vi "main.vi"() -> ()   [LabVIEW 2010]
uses:
  components_cluster.ctl
  components/Clock/GenericClock/GenericClock/GenericClock.lvclass
  components/SignalWriter/GenericSignalWriter/GenericSignalWriter/GenericSignalWriter.lvclass
  components/SignalReader/GenericSignalReader/GenericSignalReader/GenericSignalReader.lvclass
  configuration_cluster.ctl
  common/clusters/plugin_specification.ctl
  main/labview_source/type_definitions/enumerations/run_mode_enum.ctl
  <vilib>/Utility/file.llb/Write To Spreadsheet File (DBL).vi
  <vilib>/Analysis/2dsp.llb/1D Cross Correlation (DBL).vi
  common/classes/GenericComponent/GenericComponent/GenericComponent.lvclass
  <vilib>/Analysis/NI_AALPro.lvlib
panel:
  in  "normalization":enum32{"none", "unbiased", "biased"}(ring)
  in  "algorithm":enum32{"direct", "frequency domain"}(ring)
  out "phase shift":dbl[unit]
  in  "saveButton":bool
  out "cross correlation":dbl[](graph)
  in  "analyseButton":bool
  in  "channel index":i32
  out "data":dbl[](graph)
  in  "read block size":i32=16000
  in  "specifyClockButton":bool
  in  "specifyReaderButton":bool
  in  "sampling rate":dbl[unit]=20000.0
  in  "duration":dbl[unit]=1.0
  in  "specifyWriterButton":bool
  in  "stopButton":bool
  in  "startButton":bool
  in  "amplitude":dbl=1.0
  in  "frequency":dbl[unit]=10.0
  # "Amplitude and phase shift analyser"
  # "command values"
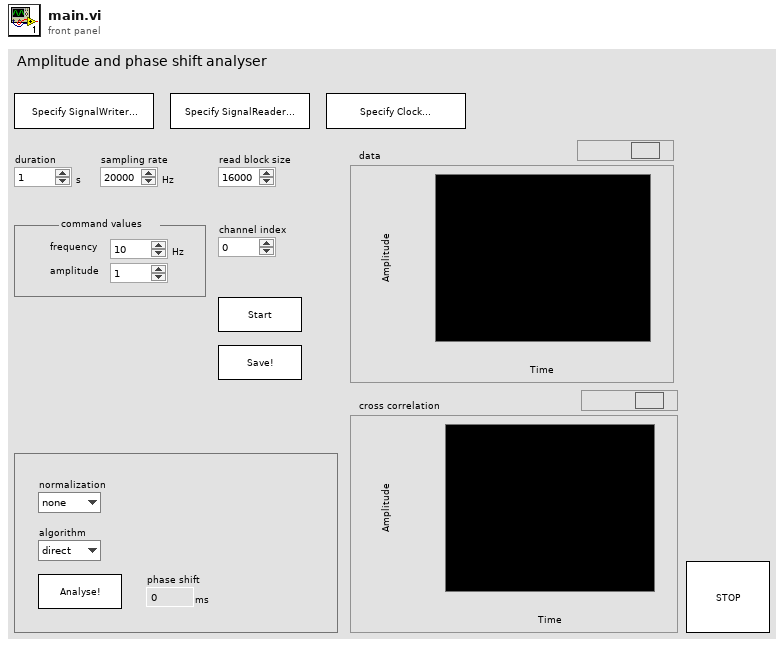
[diagram p1: front panel]
types:
  T1 = typedef "configuration_cluster.ctl" = cluster{"clock":T2, "writer":T2, "reader":T2}
  T2 = typedef "plugin_specification.ctl" = cluster{"class path":string, "configuration":string, "label":string, "settings name":string}
  T3 = typedef "components_cluster.ctl" = cluster{"clock":refnum<class "GenericClock.lvclass">, "writer":refnum<class "GenericSignalWriter.lvclass">, "reader":refnum<class "GenericSignalReader.lvclass">}
  T4 = typedef "run_mode_enum.ctl" = enum16{"focus mode", "single sweep mode", "experiment mode"}
  T5 = typedef "XComponentSpecification.xctl/data.ctl" = cluster{"class path":string, "configuration":string, "label":string, "settings name":string}
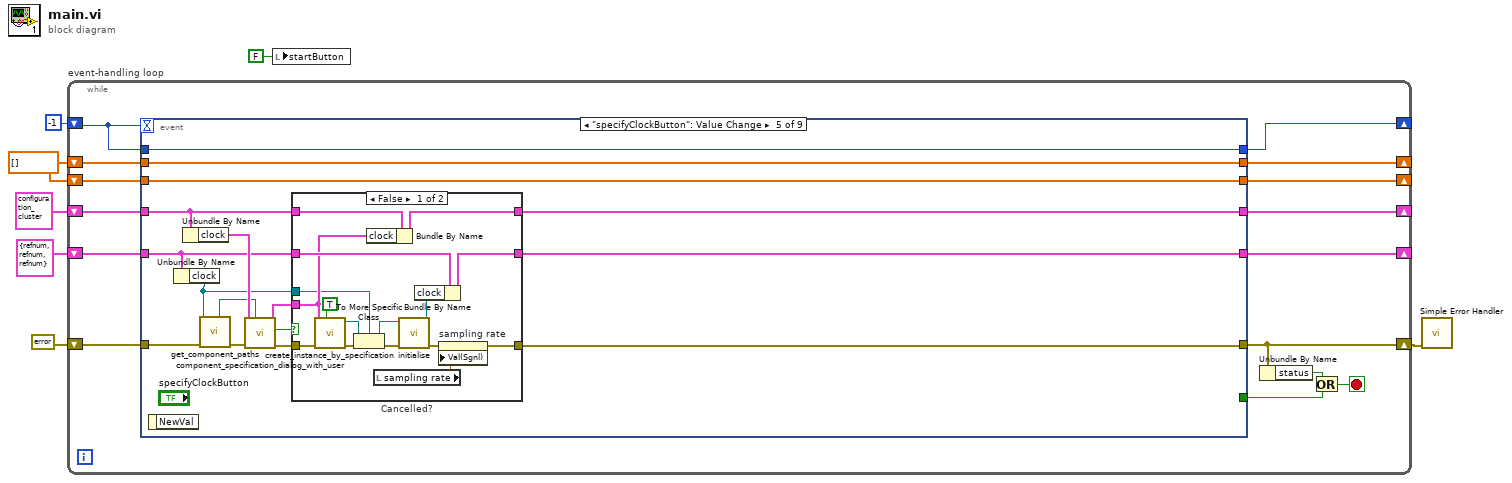
[diagram p0: block diagram]
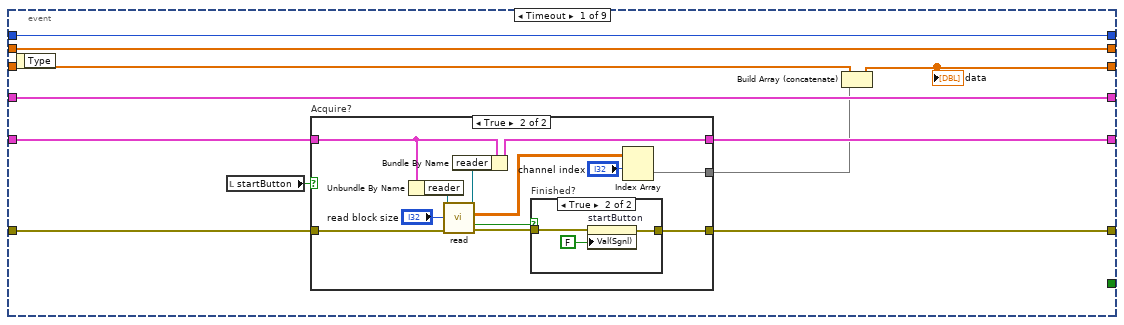
[diagram p2: hidden frame]
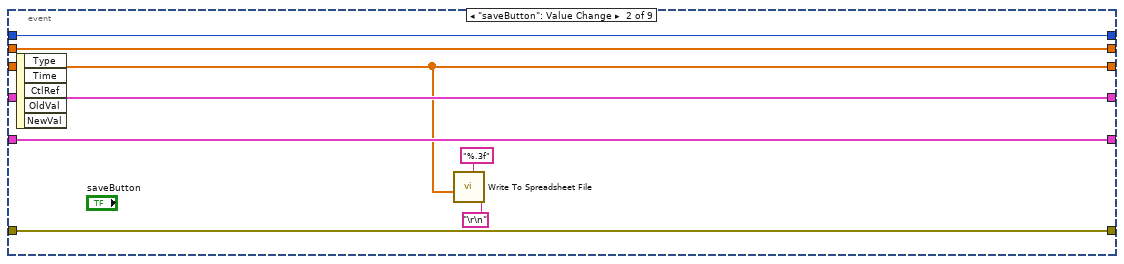
[diagram p5: hidden frame]
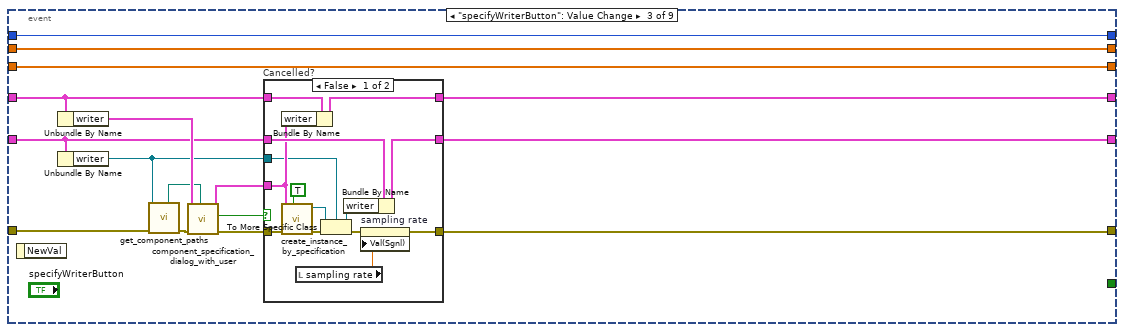
[diagram p6: hidden frame]
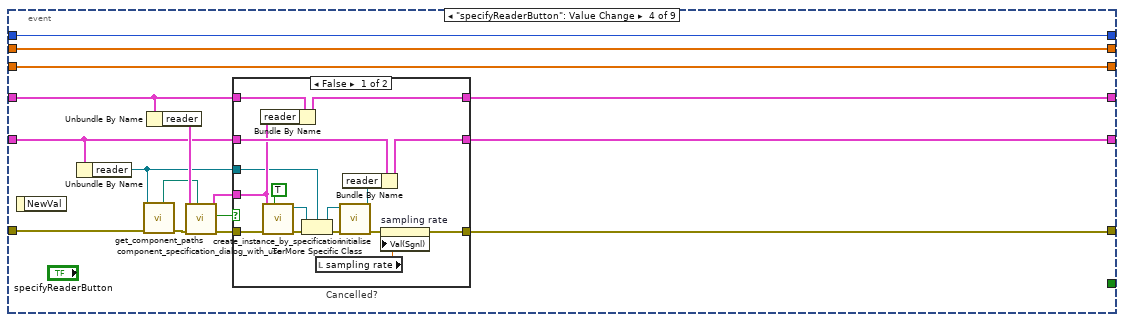
[diagram p8: hidden frame]
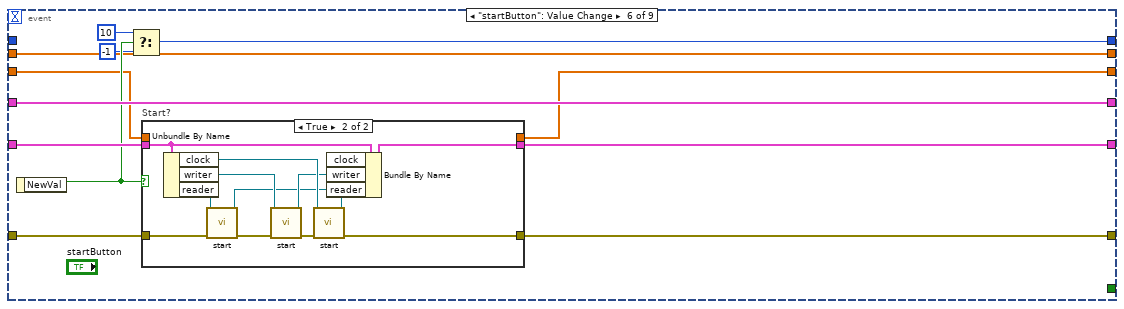
[diagram p11: hidden frame]
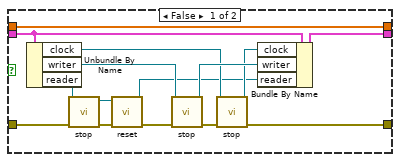
[diagram p12: hidden frame]
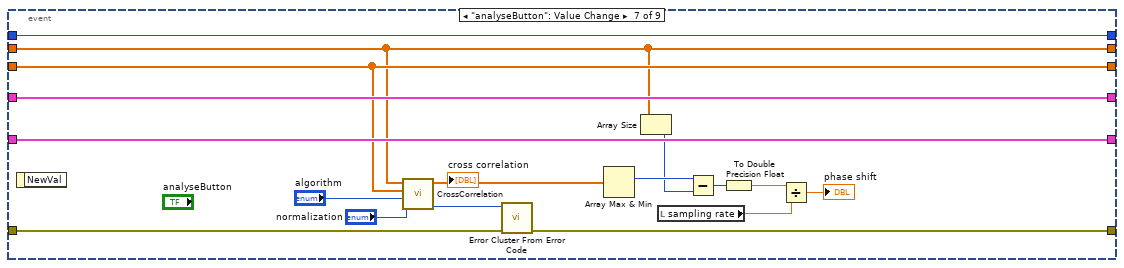
[diagram p13: hidden frame]
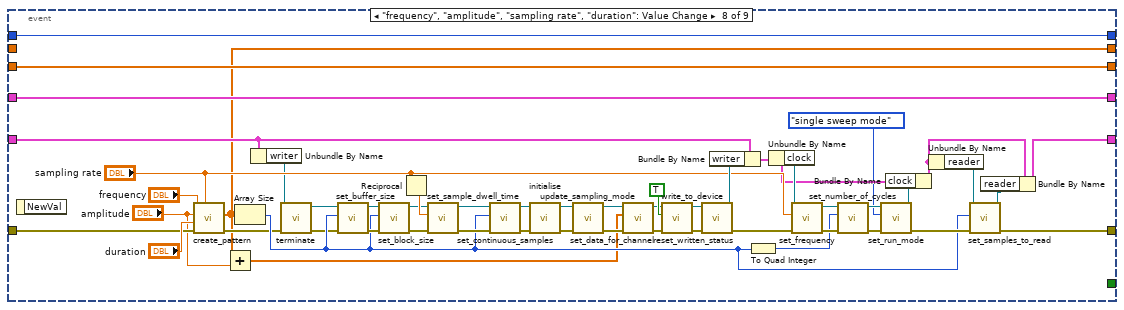
[diagram p14: hidden frame]
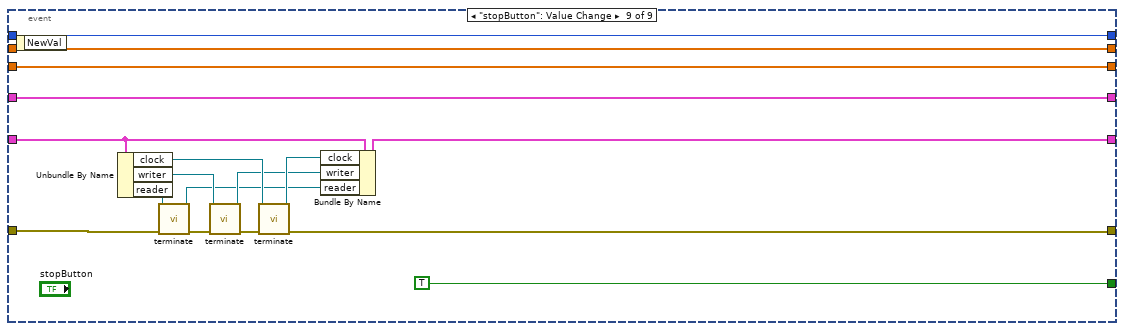
[diagram p15: hidden frame]
diagram:
  w1 = dbl[] [] ("pattern values")
  n1 = while "event-handling loop" {
    shift-right: [w21] -> w7
    shift-left: errorcluster {"status"=FALSE, "code"=0, "source"=""} ("error in (no error)") -> [w22]
    shift-right: [w16] -> _
    shift-left: T3 {"clock"=refnum, "writer"=refnum, "reader"=refnum} ("components") -> [w17]
    shift-right: [w15] -> _
    shift-left: -1 -> [w12]
    shift-right: [w13] -> _
    shift-left: T1 {"clock"={"class path"="", "configuration"="", "label"="", "settings name"=""}, "writer"={"class path"="", "configuration"="", "label"="", "settings name"=""}, "reader"={"class path"="", "configuration"="", "label"="", "settings name"=""}} ("configuration") -> [w14]
    shift-right: [w11] -> _
    shift-left: w1 -> [w10]
    shift-right: [w8] -> _
    shift-left: w1 -> [w9]
    stop <- w19 stop-if-true
    n2 = event shown="[4] \"specifyClockButton\": Value Change" {
      selector: _ -> [_ _ _ _ _ _ _ _ _]
      dyn-events: _ -> [_ _ _ _ _ _ _ _ _]
      timeout: w12 -> [_ _ _ _ _ _ _ _ _]
      tunnel: w22 -> [w30 w55 w64 w98 w132 w174 w213 w248 w284]
      tunnel: [w27 w55 w73 w104 w139 w173 w212 w237 w280] -> w21
      tunnel: [_ _ _ _ _ _ _ _ TRUE] -> w18
      tunnel: w17 -> [w32 w59 w65 w95 w131 w172 w218 w246 w277]
      tunnel: [w31 w59 w71 w103 w138 w171 w218 w233 w276] -> w16
      tunnel: [w28 w58 w75 w108 w143 w169 w211 w269 w285] -> w15
      tunnel: w14 -> [w33 w57 w69 w101 w137 w170 w217 w245 w272]
      tunnel: [w33 w57 w68 w102 w136 w170 w217 w245 w272] -> w13
      tunnel: w12 -> [w28 w58 w75 w108 w143 _ w211 w269 w285]
      tunnel: [w26 w56 w61 w94 w129 w165 w209 w221 w271] -> w11
      tunnel: w10 -> [w26 w56 w61 w94 w129 w165 w209 _ w271]
      tunnel: w9 -> [w25 w54 w60 w93 w128 w163 w216 w227 w270]
      tunnel: [w23 w54 w60 w93 w128 w164 w216 w227 w270] -> w8
      event Timeout {
        n3 = event-data() -> ()  [unwired: 1 in, 1 out]
        n4 = local read "startButton"() -> (w29:bool)
        n5 = case "Acquire?" shown="True" w29 {
          tunnel: w32 -> [w35 w46]
          tunnel: [w35 w45] -> w31
          tunnel: w30 -> [w34 w44]
          tunnel: [w34 w40] -> w27
          tunnel: [_ w36] -> w24
          frame False {
          }
          frame True {
            n6 = Unbundle By Name(w46) -> ("reader"=w43:refnum<class "GenericSignalReader.lvclass">)
            n7 = call-dynamic "read.vi"("error in (no error)"=w44, "block size"="read block size", "SignalReader in"=w43) -> ("error out"=w41:errorcluster, "finished?"=w39:bool, "signals read"=w38:dbl[][], "SignalReader out"=w47:refnum<class "GenericSignalReader.lvclass">)  [unwired: 4 in, 1 out]
            n8 = Bundle By Name(cluster=w46, "reader"=w47) -> (w45:T3)
            n9 = case "Finished?" shown="True" w39 {
              tunnel: w41 -> [w48 w51]
              tunnel: [w48 w50] -> w40
              frame False {
              }
              frame True {
                n10 = property on="startButton" class="Bool (strict)"(error in=w51, "Val(Sgnl)"=FALSE ("Value (Signaling)")) -> (error out=w50:errorcluster)  [unwired: 1 in, 1 out]
              }
            }
            n11 = Index Array(array=w38, index (row)="channel index") -> (element=w36:dbl[])  [unwired: 1 in]
          }
        }
        n12 = Build Array (concatenate)(w25, w24) -> (w23:dbl[])
        "data" <- w23
      }
      event "saveButton": Value Change {
        n13 = event-data() -> ()  [unwired: 1 in, 5 out]
        n14 = call-poly <vilib>:"Write To Spreadsheet File.vi"("delimiter (\\t)"="\r\n", "format (%.3f)"="%.3f", "1D data"=w54) -> ()  [unwired: 5 in, 1 out]
      }
      event "specifyWriterButton": Value Change {
        n15 = event-data() -> ()  [unwired: 1 in, 1 out]
        n16 = Unbundle By Name(w69) -> ("writer"=w67:T2)
        n17 = Unbundle By Name(w65) -> ("writer"=w62:refnum<class "GenericSignalWriter.lvclass">)
        n18 = call-dynamic "get_component_paths.vi"("error in (no error)"=w64, "GenericComponent in"=w62) -> ("error out"=w63:errorcluster, "component type directory"=w66:path)  [unwired: 4 in, 4 out]
        n19 = call "component_specification_dialog_with_user.vi"("start path"=w66, "error in (no error)"=w63, "component specification in"=w67) -> ("error out"=w74:errorcluster, "cancelled?"=w72:bool, "component specification out"=w70:T5)  [unwired: 6 in]
        n20 = case "Cancelled?" shown="False" w72 {
          tunnel: w74 -> [w84 w92]
          tunnel: [w88 w92] -> w73
          tunnel: [w87 w91] -> w71
          tunnel: w65 -> [w79 w91]
          tunnel: w70 -> [w77 _]
          tunnel: w69 -> [w86 w90]
          tunnel: [w85 w90] -> w68
          tunnel: w62 -> [w76 _]
          frame False {
            n21 = Bundle By Name(cluster=w86, "writer"=w77) -> (w85:T1)
            n22 = call "create_instance_by_specification.vi"("call constructor?"=TRUE, "error in (no error)"=w84, "component specification"=w77) -> ("error out"=w81:errorcluster, "GenericPlugin out"=w82:refnum<class "GenericComponent.lvclass">)  [unwired: 6 in, 1 out]
            n23 = local read "sampling rate"() -> (w89:dbl[unit])
            n24 = To More Specific Class(target class=w76, reference=w82, error in=w81) -> (specific class reference=w78:refnum<class "GenericSignalWriter.lvclass">, error out=w80:errorcluster)
            n25 = Bundle By Name(cluster=w79, "writer"=w78) -> (w87:T3)
            n26 = property on="sampling rate" class="DigNum (strict)"(error in=w80, "Val(Sgnl)"=w89) -> (error out=w88:errorcluster)  [unwired: 1 in, 1 out]
          }
          frame True {
          }
        }
      }
      event "specifyReaderButton": Value Change {
        n27 = event-data() -> ()  [unwired: 1 in, 1 out]
        n28 = Unbundle By Name(w95) -> ("reader"=w96:refnum<class "GenericSignalReader.lvclass">)
        n29 = call-dynamic "get_component_paths.vi"("error in (no error)"=w98, "GenericComponent in"=w96) -> ("error out"=w97:errorcluster, "component type directory"=w99:path)  [unwired: 4 in, 4 out]
        n30 = Unbundle By Name(w101) -> ("reader"=w100:T2)
        n31 = call "component_specification_dialog_with_user.vi"("start path"=w99, "error in (no error)"=w97, "component specification in"=w100) -> ("error out"=w105:errorcluster, "cancelled?"=w106:bool, "component specification out"=w107:T5)  [unwired: 6 in]
        n32 = case "Cancelled?" shown="False" w106 {
          tunnel: w105 -> [w117 w127]
          tunnel: [w109 w127] -> w104
          tunnel: [w123 w126] -> w103
          tunnel: w95 -> [w124 w126]
          tunnel: w107 -> [w116 _]
          tunnel: [w121 w125] -> w102
          tunnel: w101 -> [w122 w125]
          tunnel: w96 -> [w115 _]
          frame False {
            n33 = Bundle By Name(cluster=w122, "reader"=w116) -> (w121:T1)
            n34 = call "create_instance_by_specification.vi"("call constructor?"=TRUE, "error in (no error)"=w117, "component specification"=w116) -> ("error out"=w120:errorcluster, "GenericPlugin out"=w119:refnum<class "GenericComponent.lvclass">)  [unwired: 6 in, 1 out]
            n35 = To More Specific Class(target class=w115, reference=w119, error in=w120) -> (specific class reference=w113:refnum<class "GenericSignalReader.lvclass">, error out=w114:errorcluster)
            n36 = local read "sampling rate"() -> (w111:dbl[unit])
            n37 = call-dynamic "initialise.vi"("error in (no error)"=w114, "GenericPlugin in"=w113) -> ("error out"=w110:errorcluster, "GenericPlugin out"=w112:refnum<class "GenericSignalReader.lvclass">)  [unwired: 8 out]
            n38 = Bundle By Name(cluster=w124, "reader"=w112) -> (w123:T3)
            n39 = property on="sampling rate" class="DigNum (strict)"(error in=w110, "Val(Sgnl)"=w111) -> (error out=w109:errorcluster)  [unwired: 1 in, 1 out]
          }
          frame True {
          }
        }
      }
      event "specifyClockButton": Value Change {
        n40 = event-data() -> ()  [unwired: 1 in, 1 out]
        n41 = Unbundle By Name(w131) -> ("clock"=w130:refnum<class "GenericClock.lvclass">)
        n42 = Unbundle By Name(w137) -> ("clock"=w135:T2)
        n43 = call-dynamic "get_component_paths.vi"("error in (no error)"=w132, "GenericComponent in"=w130) -> ("error out"=w133:errorcluster, "component type directory"=w134:path)  [unwired: 4 in, 4 out]
        n44 = call "component_specification_dialog_with_user.vi"("start path"=w134, "error in (no error)"=w133, "component specification in"=w135) -> ("error out"=w142:errorcluster, "cancelled?"=w141:bool, "component specification out"=w140:T5)  [unwired: 6 in]
        n45 = case "Cancelled?" shown="False" w141 {
          tunnel: w142 -> [w153 w162]
          tunnel: [w144 w162] -> w139
          tunnel: [w158 w161] -> w138
          tunnel: w131 -> [w159 w161]
          tunnel: w140 -> [w151 _]
          tunnel: w137 -> [w157 w160]
          tunnel: [w156 w160] -> w136
          tunnel: w130 -> [w150 _]
          frame False {
            n46 = call "create_instance_by_specification.vi"("call constructor?"=TRUE, "error in (no error)"=w153, "component specification"=w151) -> ("error out"=w154:errorcluster, "GenericPlugin out"=w155:refnum<class "GenericComponent.lvclass">)  [unwired: 6 in, 1 out]
            n47 = To More Specific Class(target class=w150, reference=w155, error in=w154) -> (specific class reference=w148:refnum<class "GenericClock.lvclass">, error out=w149:errorcluster)
            n48 = Bundle By Name(cluster=w157, "clock"=w151) -> (w156:T1)
            n49 = local read "sampling rate"() -> (w146:dbl[unit])
            n50 = call-dynamic "initialise.vi"("error in (no error)"=w149, "GenericPlugin in"=w148) -> ("error out"=w145:errorcluster, "GenericPlugin out"=w147:refnum<class "GenericClock.lvclass">)  [unwired: 8 in]
            n51 = Bundle By Name(cluster=w159, "clock"=w147) -> (w158:T3)
            n52 = property on="sampling rate" class="DigNum (strict)"(error in=w145, "Val(Sgnl)"=w146) -> (error out=w144:errorcluster)  [unwired: 1 in, 1 out]
          }
          frame True {
          }
        }
      }
      event "startButton": Value Change {
        n53 = event-data() -> ("NewVal"=w168:bool)  [unwired: 1 in]
        n54 = Select(t=10, s=w168, f=-1) -> (s? t:f=w169:i32)
        n55 = case "Start?" shown="True" w168 {
          tunnel: w174 -> [w185 w195]
          tunnel: [w186 w190] -> w173
          tunnel: w172 -> [w183 w201]
          tunnel: [w182 w191] -> w171
          tunnel: [w175 _] -> w164
          tunnel: w163 -> [w175 _]
          frame False {
            n56 = Unbundle By Name(w183) -> ("clock"=w181:refnum<class "GenericClock.lvclass">, "writer"=w189:refnum<class "GenericSignalWriter.lvclass">, "reader"=w184:refnum<class "GenericSignalReader.lvclass">)
            n57 = call-dynamic "stop.vi"("error in (no error)"=w185, "GenericSignalReader in"=w184) -> ("error out"=w179:errorcluster, "GenericSignalReader out"=w177:refnum<class "GenericSignalReader.lvclass">)  [unwired: 8 in]
            n58 = call-dynamic "reset.vi"("error in (no error)"=w179, "GenericSignalReader in"=w177) -> ("error out"=w178:errorcluster, "GenericSignalReader out"=w176:refnum<class "GenericSignalReader.lvclass">)  [unwired: 8 in]
            n59 = call-dynamic "stop.vi"("error in (no error)"=w178, "WriteSignalsGenericPlugin in"=w189) -> ("error out"=w187:errorcluster, "WriteSignalsGenericPlugin out"=w188:refnum<class "GenericSignalWriter.lvclass">)  [unwired: 8 in]
            n60 = call-dynamic "stop.vi"("error in (no error)"=w187, "GenericClock in"=w181) -> ("error out"=w186:errorcluster, "GenericClock out"=w180:refnum<class "GenericClock.lvclass">)  [unwired: 8 in]
            n61 = Bundle By Name(cluster=w183, "clock"=w180, "writer"=w188, "reader"=w176) -> (w182:T3)
          }
          frame True {
            n62 = Unbundle By Name(w201) -> ("clock"=w199:refnum<class "GenericClock.lvclass">, "writer"=w197:refnum<class "GenericSignalWriter.lvclass">, "reader"=w196:refnum<class "GenericSignalReader.lvclass">)
            n63 = call-dynamic "start.vi"("error in (no error)"=w195, "GenericSignalReader in"=w196) -> ("error out"=w194:errorcluster, "GenericSignalReader out"=w192:refnum<class "GenericSignalReader.lvclass">)  [unwired: 8 in]
            n64 = call-dynamic "start.vi"("error in (no error)"=w194, "WriteSignalsGenericPlugin in"=w197) -> ("error out"=w200:errorcluster, "WriteSignalsGenericPlugin out"=w198:refnum<class "GenericSignalWriter.lvclass">)  [unwired: 8 in]
            n65 = call-dynamic "start.vi"("error in (no error)"=w200, "GenericClock in"=w199) -> ("error out"=w190:errorcluster, "GenericClock out"=w193:refnum<class "GenericClock.lvclass">)  [unwired: 8 in]
            n66 = Bundle By Name(cluster=w201, "clock"=w193, "writer"=w198, "reader"=w192) -> (w191:T3)
          }
        }
      }
      event "analyseButton": Value Change {
        n67 = event-data() -> ()  [unwired: 1 in, 1 out]
        n68 = call-poly <vilib>:"CrossCorrelation.vi"("normalization"="normalization", "algorithm"="algorithm", "Y"=w216, "X"=w209) -> ("error"=w214:i32, "Rxy"=w210:dbl[])  [unwired: 6 in]
        "cross correlation" <- w210
        n69 = call <vilib>:"Error Cluster From Error Code.vi"("error in (no error)"=w213, "error code (0)"=w214) -> ("error out"=w212:errorcluster)  [unwired: 7 in]
        n70 = Array Max & Min(array=w210) -> (max index (indices)=w208:i32)  [unwired: 3 out]
        n71 = Array Size(array=w209) -> (size(s)=w207:i32)
        n72 = local read "sampling rate"() -> (w204:dbl[unit])
        n73 = Subtract(x=w208, y=w207) -> (x-y=w206:i32)
        n74 = To Double Precision Float(number=w206) -> (double precision float=w205:dbl)
        n75 = Divide(x=w205, y=w204) -> (x/y=→"phase shift":dbl[unit])
      }
      event "frequency", "amplitude", "sampling rate", "duration": Value Change {
        n76 = event-data() -> ()  [unwired: 1 in, 1 out]
        n77 = call "create_pattern.vi"("sampling rate"="sampling rate", "error in (no error)"=w248, "duration"="duration", "amplitude"="amplitude", "frequency"="frequency") -> ("error out"=w224:errorcluster, "pattern values"=w221:dbl[])  [unwired: 5 in]
        n78 = Add(x=w221, y="amplitude") -> (x+y=w220:dbl[])
        n79 = Array Size(array=w221) -> (size(s)=w226:i32)
        n80 = Unbundle By Name(w246) -> ("writer"=w223:refnum<class "GenericSignalWriter.lvclass">)
        n81 = call-dynamic "terminate.vi"("error in (no error)"=w224, "GenericPlugin in"=w223) -> ("error out"=w225:errorcluster, "GenericPlugin out"=w222:refnum<class "GenericSignalWriter.lvclass">)  [unwired: 8 in]
        n82 = call-dynamic "set_buffer_size.vi"("error in (no error)"=w225, "buffer size (samples)"=w226, "GenericWriteSignals.lvclass in"=w222) -> ("error out"=w249:errorcluster, "GenericWriteSignals.lvclass out"=w250:refnum<class "GenericSignalWriter.lvclass">)  [unwired: 7 out]
        n83 = call "set_block_size.vi"("error in (no error)"=w249, "block size (samples)"=w226, "GenericWriteSignals.lvclass in"=w250) -> ("error out"=w251:errorcluster, "GenericWriteSignals.lvclass out"=w252:refnum<class "GenericSignalWriter.lvclass">)  [unwired: 7 in]
        n84 = Reciprocal(x="sampling rate") -> (1/x=w264:dbl[unit])
        n85 = call-dynamic "set_sample_dwell_time.vi"("error in (no error)"=w251, "sample dwell time"=w264, "GenericWriteSignals.lvclass in"=w252) -> ("error out"=w255:errorcluster, "GenericWriteSignals.lvclass out"=w258:refnum<class "GenericSignalWriter.lvclass">)  [unwired: 7 in]
        n86 = call-dynamic "set_continuous_samples.vi"("error in (no error)"=w255, "continuous samples"=w226, "GenericWriteSignals.lvclass in"=w258) -> ("error out"=w256:errorcluster, "GenericWriteSignals.lvclass out"=w257:refnum<class "GenericSignalWriter.lvclass">)  [unwired: 7 out]
        n87 = call-dynamic "initialise.vi"("error in (no error)"=w256, "GenericPlugin in"=w257) -> ("error out"=w253:errorcluster, "GenericPlugin out"=w254:refnum<class "GenericSignalWriter.lvclass">)  [unwired: 8 out]
        n88 = call-dynamic "update_sampling_mode.vi"("error in (no error)"=w253, "GenericWriteSignals in"=w254) -> ("error out"=w259:errorcluster, "GenericWriteSignals out"=w262:refnum<class "GenericSignalWriter.lvclass">)  [unwired: 8 out]
        n89 = call-dynamic "set_data_for_channel.vi"("error in (no error)"=w259, "data"=w220, "GenericWriteSignals in"=w262) -> ("error out"=w260:errorcluster, "GenericWriteSignals out"=w261:refnum<class "GenericSignalWriter.lvclass">)  [unwired: 7 out]
        n90 = call-dynamic "write_to_device.vi"("error in (no error)"=w260, "force writing?"=TRUE, "GenericWriteSignals in"=w261) -> ("error out"=w265:errorcluster, "GenericWriteSignals out"=w266:refnum<class "GenericSignalWriter.lvclass">)  [unwired: 7 out]
        n91 = call-dynamic "reset_written_status.vi"("error in (no error)"=w265, "GenericWriteSignals in"=w266) -> ("error out"=w244:errorcluster, "GenericWriteSignals out"=w247:refnum<class "GenericSignalWriter.lvclass">)  [unwired: 8 out]
        n92 = Bundle By Name(cluster=w246, "writer"=w247) -> (w239:T3)
        n93 = To Quad Integer(1:w226) -> (0:w238:i64)
        n94 = Unbundle By Name(w239) -> ("clock"=w240:refnum<class "GenericClock.lvclass">)
        n95 = call-dynamic "set_frequency.vi"("error in (no error)"=w244, "frequency"="sampling rate", "GenericClock.lvclass in"=w240) -> ("error out"=w243:errorcluster, "GenericClock.lvclass out"=w242:refnum<class "GenericClock.lvclass">)  [unwired: 7 in]
        n96 = call-dynamic "set_number_of_cycles.vi"("error in (no error)"=w243, "number of cycles"=w238, "GenericClock.lvclass in"=w242) -> ("error out"=w232:errorcluster, "GenericClock.lvclass out"=w229:refnum<class "GenericClock.lvclass">)  [unwired: 7 in]
        n97 = call-dynamic "set_run_mode.vi"("error in (no error)"=w232, "run mode"=run_mode_enum."single sweep mode", "GenericPlugin in"=w229) -> ("error out"=w231:errorcluster, "GenericPlugin out"=w230:refnum<class "GenericClock.lvclass">)  [unwired: 7 in]
        n98 = Bundle By Name(cluster=w239, "clock"=w230) -> (w234:T3)
        n99 = Unbundle By Name(w234) -> ("reader"=w236:refnum<class "GenericSignalReader.lvclass">)
        n100 = call-dynamic "set_samples_to_read.vi"("error in (no error)"=w231, "samples to read"=w226, "GenericSignalReader in"=w236) -> ("error out"=w237:errorcluster, "GenericSignalReader out"=w235:refnum<class "GenericSignalReader.lvclass">)  [unwired: 7 in]
        n101 = Bundle By Name(cluster=w234, "reader"=w235) -> (w233:T3)
      }
      event "stopButton": Value Change {
        n102 = event-data() -> ()  [unwired: 1 in, 1 out]
        n103 = Unbundle By Name(w277) -> ("clock"=w278:refnum<class "GenericClock.lvclass">, "writer"=w279:refnum<class "GenericSignalWriter.lvclass">, "reader"=w283:refnum<class "GenericSignalReader.lvclass">)
        n104 = call-dynamic "terminate.vi"("error in (no error)"=w284, "GenericPlugin in"=w283) -> ("error out"=w281:errorcluster, "GenericPlugin out"=w273:refnum<class "GenericSignalReader.lvclass">)  [unwired: 8 in]
        n105 = call-dynamic "terminate.vi"("error in (no error)"=w281, "GenericPlugin in"=w279) -> ("error out"=w282:errorcluster, "GenericPlugin out"=w274:refnum<class "GenericSignalWriter.lvclass">)  [unwired: 8 in]
        n106 = call-dynamic "terminate.vi"("error in (no error)"=w282, "GenericPlugin in"=w278) -> ("error out"=w280:errorcluster, "GenericPlugin out"=w275:refnum<class "GenericClock.lvclass">)  [unwired: 8 in]
        n107 = Bundle By Name(cluster=w277, "clock"=w275, "writer"=w274, "reader"=w273) -> (w276:T3)
      }
    }
    n108 = Unbundle By Name(w21) -> ("status"=w20:bool)
    n109 = Or(x=w20, y=w18) -> (x .or. y?=w19:bool)
  }
  n110 = local write "startButton"(FALSE ("startButton")) -> ()
  n111 = call <vilib>:"Simple Error Handler.vi"("error in (no error)"=w7) -> ()  [unwired: 4 in, 5 out]
